vi "Add Delay.vi"(8 "error in (no error)":errorcluster, 9 "# Samples":i32, 11 "I2C waveform info":T1) -> (0 "error out":errorcluster, 3 "I2C waveform info out":T1)   [LabVIEW 2009, in "IDW.lvlib"]
doc: "Adds a delay to the I2C waveform, wherein the states of both bus lines (SCL, SDA) are not changed. The length of the delay is determined by the <b># Samples</b> control, whose units are ticks of the sample clock. For example, an input of '4' will append four samples to the waveform."
uses:
  IDW.lvlib
  _Typedefs/Waveform info.ctl
  _Typedefs/Timing - ticks.ctl
  _Typedefs/Default transition action.ctl
  _Typedefs/Bit type.ctl
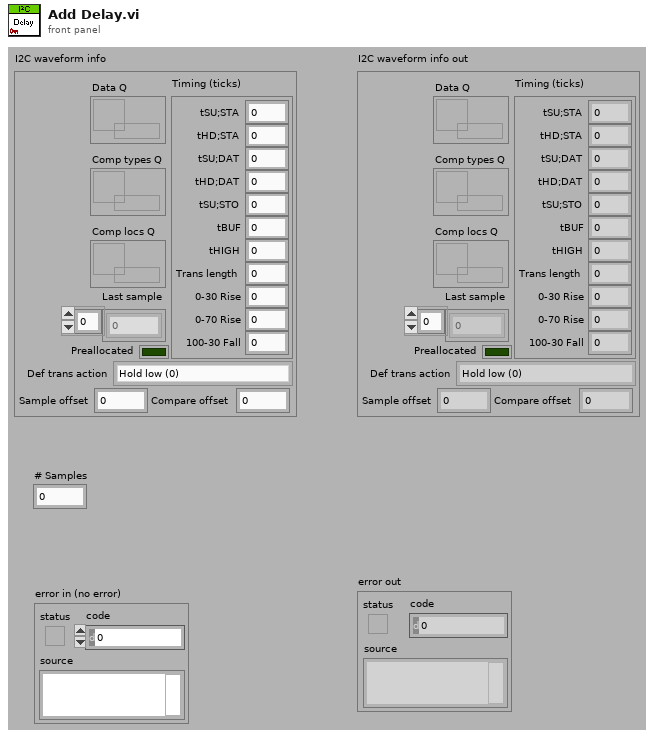
[diagram p1: front panel]
types:
  T1 = typedef "IDW.lvlib/Waveform info.ctl" = cluster{"Last sample":u8[], "Sample offset":u64, "Compare offset":u64, "Timing (ticks)":T2, "Preallocated":bool, "Def trans action":T3, "Data Q":refnum<queue>, "Comp types Q":refnum<queue>, "Comp locs Q":refnum<queue>}
  T2 = typedef "IDW.lvlib/Timing - ticks.ctl" = cluster{"tSU;STA":i32, "tHD;STA":i32, "tSU;DAT":i32, "tHD;DAT":i32, "tSU;STO":i32, "tBUF":i32, "tHIGH":i32, "Trans length":i32, "0-30 Rise":i32, "0-70 Rise":i32, "100-30 Fall":i32}
  T3 = typedef "IDW.lvlib/Default transition action.ctl" = enum16{"Hold low (0)", "Release (Z)", "Set up next value", "Hold previous value", "Preserve tHD;DAT and tSU;DAT"}
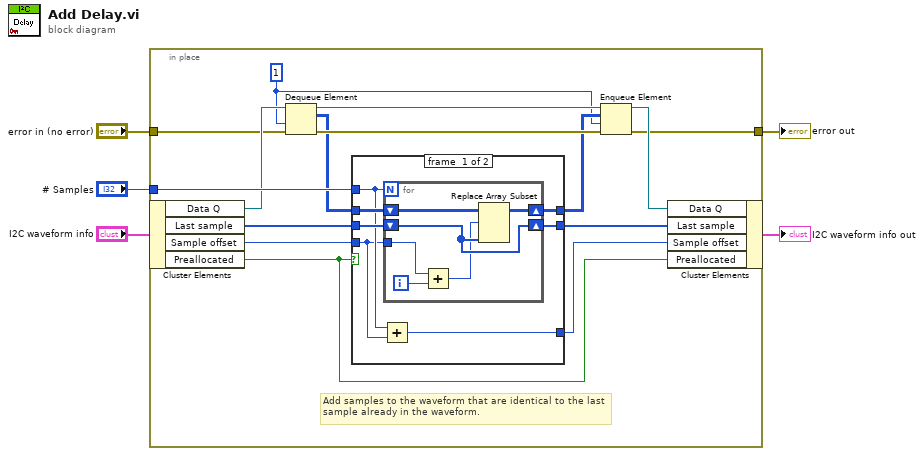
[diagram p0: block diagram]
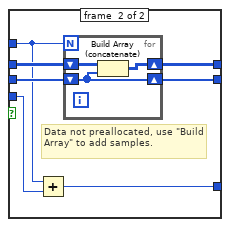
[diagram p2: hidden frame]
diagram:
  n1 = in-place {
    in-place-border: "# Samples" -> [w18]
    in-place-border: "error in (no error)" -> [w7]
    in-place-border: [w6] -> w1
    w9 = 1 ("timeout in ms (-1)")
    # "Add samples to the waveform that are identical to the last sample already in the waveform."
    n2 = in-place-cluster #1("I2C waveform info") -> ("Data Q"=w14:refnum<queue>, "Last sample"=w20:u8[], "Sample offset"=w16:u64, "Preallocated"=w17:bool)
    n3 = Dequeue Element(queue=w14, timeout in ms (-1)=w9, error in (no error)=w7) -> (queue out=w13:refnum<queue>, element=w10:u8[][], error out=w12:errorcluster)  [unwired: 1 out]
    n4 = case shown="True" w17 {
      tunnel: w20 -> [w27 w40]
      tunnel: [w26 w39] -> w19
      tunnel: w18 -> [w23 w36]
      tunnel: w10 -> [w25 w38]
      tunnel: [w24 w37] -> w11
      tunnel: w16 -> [w22 w35]
      tunnel: [w21 w34] -> w15
      frame #0 {
        n5 = Add(x=w23, y=w22) -> (x+y=w21:u64)
        n6 = for {
          N: w23 -> [_]
          shift-right: [w32] -> w24
          shift-left: w25 -> [w33]
          shift-right: [w31] -> w26
          shift-left: w27 -> [w31]
          tunnel: w22 -> [w28]
          i -> [w30]
          n7 = Add(x=w28, y=w30) -> (x+y=w29:u64)
          n8 = Replace Array Subset(array=w33, new element=w31, index (row)=w29) -> (w32:u8[][])  [unwired: 1 in]
        }
      }
      frame #1 {
        # "Data not preallocated, use \"Build Array\" to add samples."
        n9 = Add(x=w36, y=w35) -> (x+y=w34:u64)
        n10 = for {
          N: w36 -> [_]
          shift-right: [w42] -> w37
          shift-left: w38 -> [w43]
          shift-right: [w41] -> w39
          shift-left: w40 -> [w41]
          n11 = Build Array (concatenate)(w43, w41) -> (w42:u8[][])
        }
      }
    }
    n12 = Enqueue Element(queue=w13, element=w11, timeout in ms (-1)=w9, error in (no error)=w12) -> (queue out=w8:refnum<queue>, error out=w6:errorcluster)  [unwired: 1 out]
    n13 = in-place-cluster #1("Data Q"=w8, "Last sample"=w19, "Sample offset"=w15, "Preallocated"=w17) -> (→"I2C waveform info out":T1)
  }
  "error out" <- w1
